vi "test_Create Global MetaData Channel_array type cast.vi"(8 "error in (no error)":errorcluster, 11 "TestCase in":refnum<class "Instrument Addon Scripting API Channels Unit Tests.lvclass">) -> (0 "error out":errorcluster, 3 "TestCase out":refnum<class "Instrument Addon Scripting API Channels Unit Tests.lvclass">)   [LabVIEW 2018, in "Instrument Addon Scripting API Channels Unit Tests.lvclass"]
uses:
  Instrument Addon Scripting API Channels Unit Tests.lvclass
  Addon/Addon Shared/Types/FG Control.ctl
  APIs/Scripting API/TypeDefs/Array Type Cast Settings.ctl
  APIs/Scripting API/TypeDefs/Array Element.ctl
  Addon/Addon Shared/Types/Type Cast Type.ctl
  Addon/Addon Shared/Types/Endian.ctl
  Instrument Addon Scripting API Channels Unit Tests.lvclass/Instrument Addon Scripting API Channels Unit Tests.ctl
  Addon/Addon Shared/SubVIs/Constants.vi
  APIs/Scripting API/Channels/Create Global MetaData Channel - Array - Type Cast.vi
  <vilib>/NI Veristand/Custom Device Tools/Custom Device Utility Library/NI VeriStand - Search for Item by GUID.vi
  <vilib>/NI Veristand/Custom Device Tools/Custom Device Utility Library/NI VeriStand - Search for Item by Name.vi
  <vilib>/NI Veristand/Custom Device API/NI VeriStand - Get Item Property.vi
  <vilib>/NI Veristand/Custom Device API/Get Item Property (U32).vi
  <vilib>/NI Veristand/Custom Device API/Get Item Property (String Array).vi
  <vilib>/NI Veristand/Custom Device API/Get Item Property (String).vi
  <vilib>/NI Veristand/Custom Device API/NI VeriStand - Set Item Property.vi
  <vilib>/NI Veristand/Custom Device API/Set Item Property (U32).vi
  <vilib>/NI Veristand/Custom Device API/Set Item Property (String Array).vi
  <vilib>/NI Veristand/Custom Device API/NI VeriStand - Get Item Children.vi
  Addon/Addon Shared/SubVIs/Set Channel Value Table.vi
  <vilib>/NI Veristand/Custom Device API/Set Item Property (String).vi
  <vilib>/addons/_JKI Toolkits/VI Tester/TestCase.llb/TestCase.lvclass
  Instrument Addon Scripting API Test Assets/Instrument Addon Scripting API Test Assets.lvclass
  <vilib>/NI Veristand/Custom Device Tools/Custom Device Utility Library/Custom Device Utility Library.lvlib
  Addon/Addon Shared/Instrument Addon Shared.lvlib
  APIs/Scripting API/Instrument Addon Scripting API.lvlib
  C:/Program Files (x86)/National Instruments/LabVIEW 2018/vi.lib/addons/_JKI Toolkits/VI Tester/TestCase.llb/TestCase.lvclass
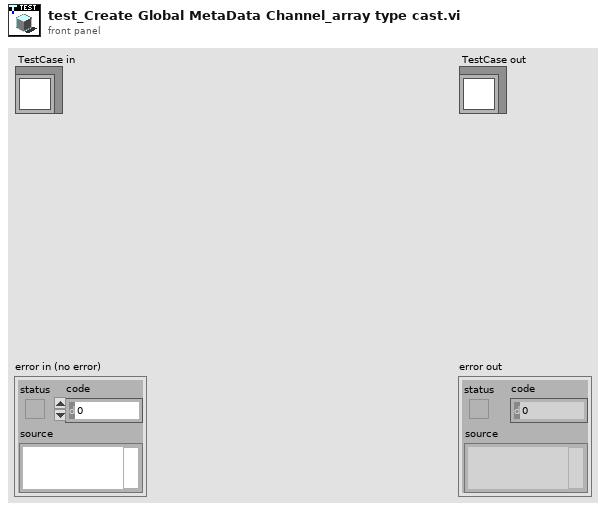
[diagram p1: front panel]
types:
  T1 = typedef "Instrument Addon Shared.lvlib/FG Control.ctl" = enum16{"Get", "Set"}
  T2 = typedef "Instrument Addon Scripting API.lvlib/Array Type Cast Settings.ctl" = cluster{"Elements":T3[], "Type":T4, "Endian":T5, "Delimiter":string}
  T3 = typedef "Instrument Addon Scripting API.lvlib/Array Element.ctl" = cluster{"Name":string, "Default Value":dbl, "Units":string}
  T4 = typedef "Instrument Addon Shared.lvlib/Type Cast Type.ctl" = enum16{"DBL", "SGL", "U64", "U32", "U16", "U8", "I64", "I32", "I16", "I8"}
  T5 = typedef "Instrument Addon Shared.lvlib/Endian.ctl" = enum16{"Native", "Little", "Big"}
  T6 = typedef "Custom Device API.lvlib/Custom Device Item Ref.ctl" = u64
  T7 = typedef "Instrument Addon Shared.lvlib/MetaData Parameters.ctl" = cluster{"Data Type":T8, "Channel Type":T9, "List":string[], "Format String":string, "Type":T4, "Delimiter":string, "Endian":T5}
  T8 = typedef "Instrument Addon Shared.lvlib/Protocol Data Type.ctl" = enum16{"Single Channel", "Array"}
  T9 = typedef "Instrument Addon Shared.lvlib/Metadata Channel Type.ctl" = enum16{"Enumerated List", "Format", "Type Cast"}
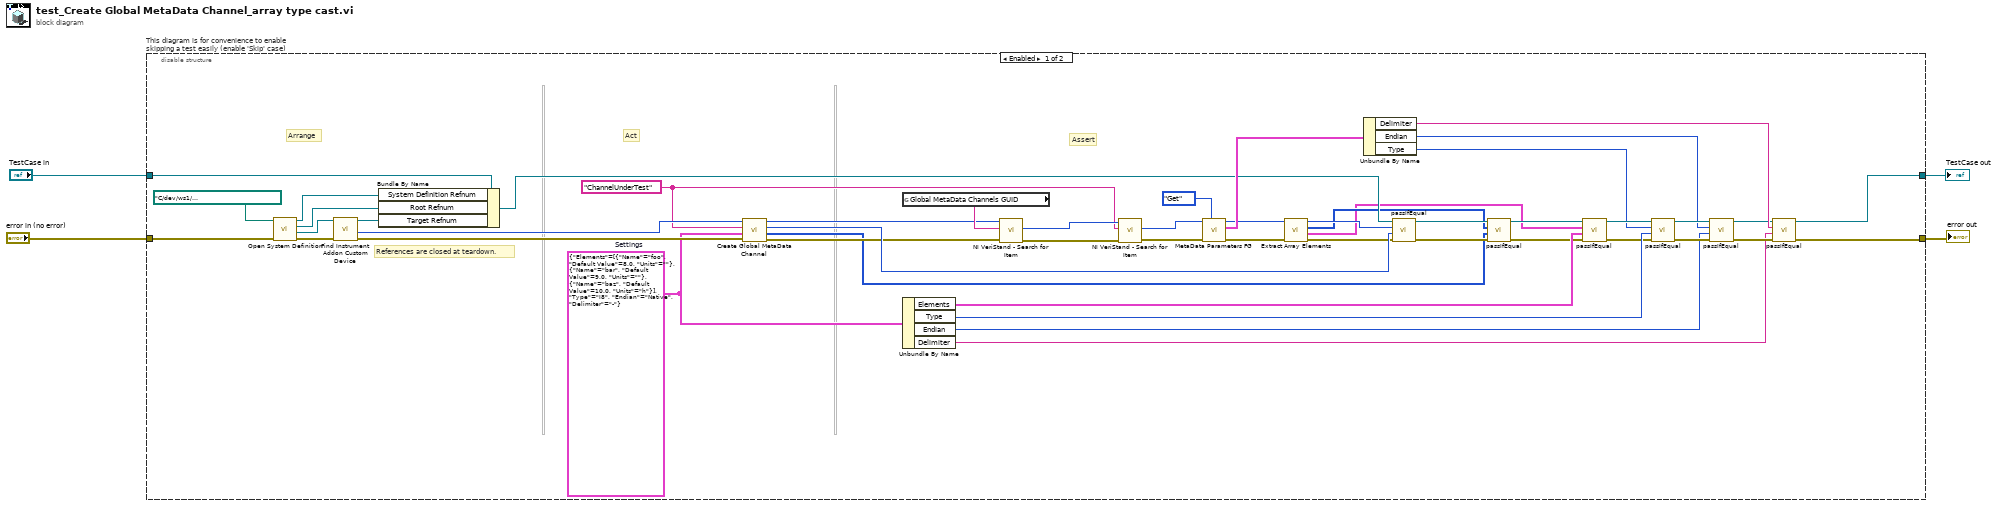
[diagram p0: block diagram]
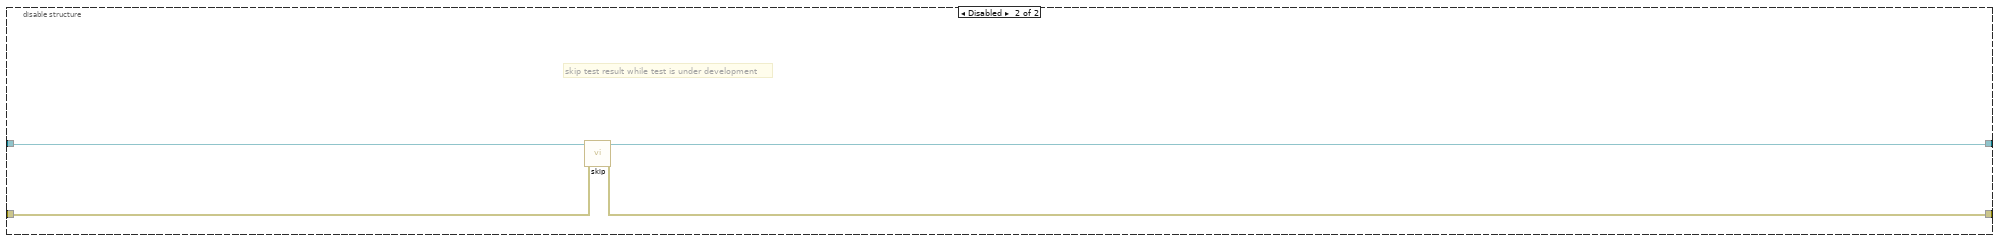
[diagram p2: hidden frame]
diagram:
  n1 = disable-structure "This diagram is for convenience to enable skipping a test easily (enable 'Skip' case)" shown="Enabled" {
    disable-tunnel: "TestCase in" -> [w37 w57]
    disable-tunnel: [w29 w55] -> w1
    disable-tunnel: [w28 w56] -> w3
    disable-tunnel: "error in (no error)" -> [w53 w54]
    frame Enabled {
      w20 = T2 {"Elements"=[{"Name"="foo", "Default Value"=8.0, "Units"=""}, {"Name"="bar", "Default Value"=9.0, "Units"=""}, {"Name"="baz", "Default Value"=10.0, "Units"="h"}], "Type"=enum."I8", "Endian"=enum."Native", "Delimiter"="-"}  # Settings
      w35 = "ChannelUnderTest" ("Name")
      # "References are closed at teardown."
      # "Assert"
      # "Act"
      # "Arrange"
      n2 = call "Open System Definition.vi"("error in (no error)"=w53, "System Definition File"=path "C:/dev/ws1/niveristand-instrument-addon-custom-device/Source/Tests/Unit Tests/Scripting API/Instrument Addon Scripting API Channels Unit Tests/Assets/MetaData Channels/IACD_channels.nivssdf") -> ("error out"=w51:errorcluster, "Target Refnum"=w52:refnum<k24>, "Root Refnum"=w40:refnum<k24>, "System Definition Refnum"=w39:refnum<k24>)  [unwired: 6 in]
      n3 = call "Find Instrument Addon Custom Device.vi"("error in"=w51, "target in"=w52) -> ("error out"=w34:errorcluster, "NodeID"=w36:u64, "target out"=w41:refnum<k24>)  [unwired: 7 in]
      n4 = Bundle By Name(cluster=w37, "System Definition Refnum"=w39, "Root Refnum"=w40, "Target Refnum"=w41) -> (w38:refnum<class "Instrument Addon Scripting API Channels Unit Tests.lvclass">)
      n5 = call-poly "Create Global MetaData Channel.vi"("Error In"=w34, "Settings"=w20, "Name"=w35, "Instrument Addon Refnum In"=w36) -> ("Error Out"=w31:errorcluster, "Channel Refnums"=w5:T6[], "Array Refnum"=w32:T6, "Instrument Addon Refnum Out"=w33:T6)  [unwired: 4 in]
      n6 = global read "Constants.vi" "Global MetaData Channels GUID"() -> (w49:string)
      n7 = Unbundle By Name(w20) -> ("Elements"=w25:T3[], "Type"=w42:T4, "Endian"=w15:T5, "Delimiter"=w12:string)
      n8 = call-poly <vilib>:"NI VeriStand - Search for Item.vi"("error in"=w31, "Item GUID"=w49, "Section Ref in"=w33) -> ("error out"=w47:errorcluster, "Item Ref"=w48:T6)  [unwired: 5 in, 2 out]
      n9 = call-poly <vilib>:"NI VeriStand - Search for Item.vi"("error in"=w47, "Item Name"=w35, "Section Ref in"=w48) -> ("error out"=w46:errorcluster, "Item Ref"=w45:T6)  [unwired: 5 in, 2 out]
      n10 = call "MetaData Parameters FG.vi"("Action"=FG_Control."Get", "error in (no error)"=w46, "Item Ref in"=w45) -> ("error out"=w24:errorcluster, "MetaData Parameters"=w43:T7, "Item Ref out"=w23:T6)  [unwired: 6 in]
      n11 = call "Extract Array Elements.vi"("error in (no error)"=w24, "array reference in"=w23) -> ("error out"=w22:errorcluster, "elements"=w6:T3[], "channel refnums"=w7:T6[], "array reference out"=w21:T6)  [unwired: 6 in]
      n12 = Unbundle By Name(w43) -> ("Delimiter"=w30:string, "Endian"=w13:T5, "Type"=w14:T4)
      n13 = call-dynamic "passIfEqual.vi"("error in (no error)"=w22, "y"=w32, "x"=w21, "TestCase in"=w38) -> ("error out"=w9:errorcluster, "TestCase out"=w11:refnum<class "Instrument Addon Scripting API Channels Unit Tests.lvclass">)  [unwired: 6 in]
      n14 = call-dynamic "passIfEqual.vi"("error in (no error)"=w9, "y"=w5, "x"=w7, "TestCase in"=w11) -> ("error out"=w8:errorcluster, "TestCase out"=w10:refnum<class "Instrument Addon Scripting API Channels Unit Tests.lvclass">)  [unwired: 6 in]
      n15 = call-dynamic "passIfEqual.vi"("error in (no error)"=w8, "y"=w25, "x"=w6, "TestCase in"=w10) -> ("error out"=w26:errorcluster, "TestCase out"=w27:refnum<class "Instrument Addon Scripting API Channels Unit Tests.lvclass">)  [unwired: 6 in]
      n16 = call-dynamic "passIfEqual.vi"("error in (no error)"=w26, "y"=w42, "x"=w14, "TestCase in"=w27) -> ("error out"=w18:errorcluster, "TestCase out"=w19:refnum<class "Instrument Addon Scripting API Channels Unit Tests.lvclass">)  [unwired: 6 in]
      n17 = call-dynamic "passIfEqual.vi"("error in (no error)"=w18, "y"=w15, "x"=w13, "TestCase in"=w19) -> ("error out"=w16:errorcluster, "TestCase out"=w17:refnum<class "Instrument Addon Scripting API Channels Unit Tests.lvclass">)  [unwired: 6 in]
      n18 = call-dynamic "passIfEqual.vi"("error in (no error)"=w16, "y"=w12, "x"=w30, "TestCase in"=w17) -> ("error out"=w28:errorcluster, "TestCase out"=w29:refnum<class "Instrument Addon Scripting API Channels Unit Tests.lvclass">)  [unwired: 6 in]
    }
    frame Disabled {
      # "skip test result while test is under development"
      n19 = call <vilib>:"skip.vi"("error in (no error)"=w54, "TestCase in"=w57) -> ("error out"=w56:errorcluster, "TestCase out"=w55:refnum<class "Instrument Addon Scripting API Channels Unit Tests.lvclass">)  [unwired: 8 in]
    }
  }
  "error out" <- w3
  "TestCase out" <- w1
